vi "_Run Cycle Param.vi"(1 "Init (F)":bool) -> (0 "Finish Run?":bool)   [LabVIEW 2012]
uses:
  <vilib>/rvi/DataTransferAndStorage/Container/Common/niFpgaContainerGetUniqueNameForEmu.vi
  <vilib>/rvi/Memory/Memory_Emulation/niFpgaMemoryEmulationCacheClearOnFirstRun.vi
  <vilib>/rvi/Memory/Memory_Emulation/nirvimemoryEmulationManagerCache_MakeExclusive.vi
  <vilib>/rvi/Memory/Memory_Emulation/niFpgaMemoryEmulationValidateCache.vi
  <vilib>/rvi/Memory/Memory_Emulation/nirvimemoryEmulationManagerCache_ReleaseExclusive.vi
  <vilib>/rvi/Memory/Memory_Emulation/nirvimemoryEmulationManagerCache_InsertValue.vi
  <vilib>/Utility/error.llb/Clear Errors.vi
  <vilib>/rvi/Memory/Memory_Emulation/nirvimemoryEmulationManagerCache_GetValue.vi
  <vilib>/rvi/Emulation/niFpgaSctlEmulationGetInTimedLoop.vi
  <vilib>/rvi/Memory/Memory_Emulation/nirvimemoryEmulationManagerCache_SetValue.vi
  <vilib>/rvi/Emulation/niFpgaSctlEmulationResourceMgr.vi
  Instance           9 18Saved   _Run Cycle .vi
  <vilib>/rvi/DataTransferAndStorage/Container/XNode/niFpgaContainer.xnode
  <vilib>/rvi/Memory/Memory_Emulation/nirvimemoryEmulation.vi
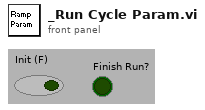
[diagram p1: front panel]
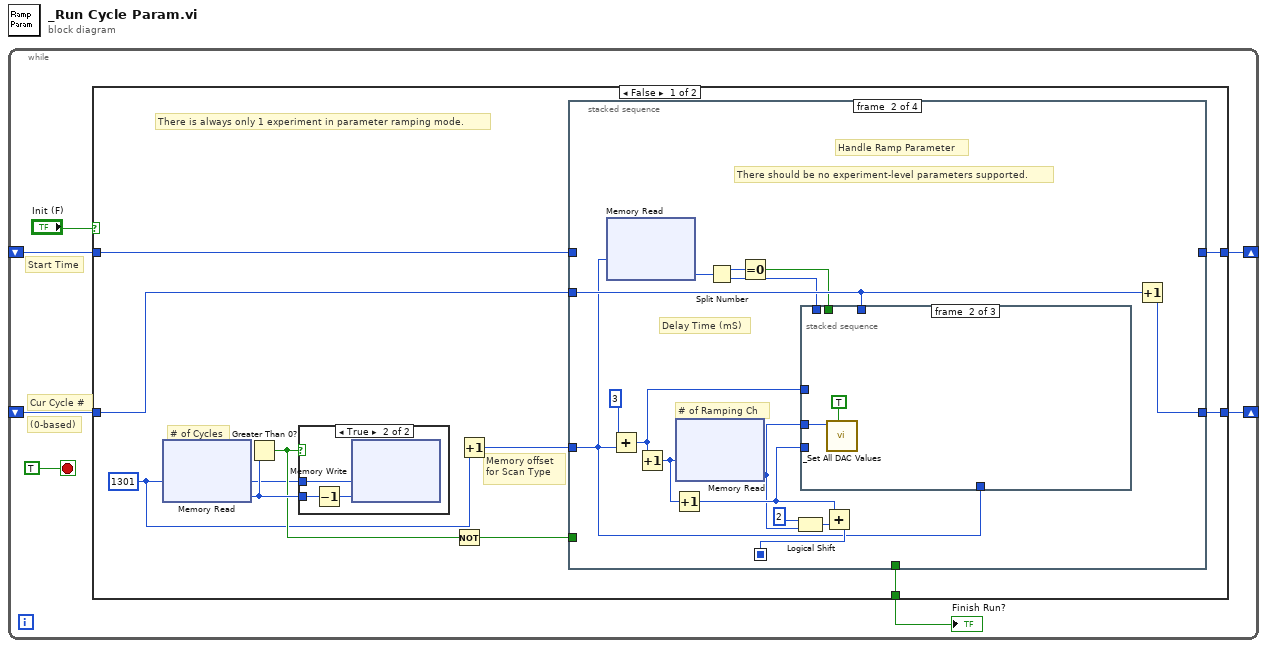
[diagram p0: block diagram]
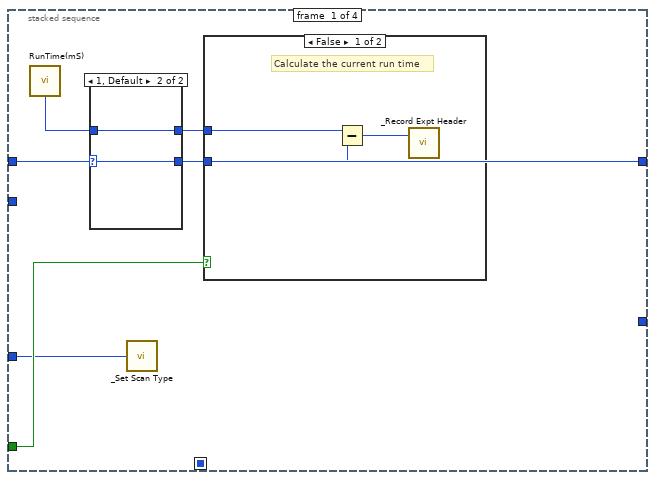
[diagram p3: hidden frame]
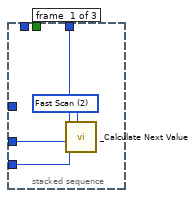
[diagram p6: hidden frame]
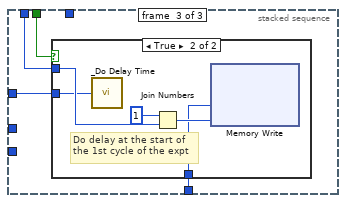
[diagram p7: hidden frame]
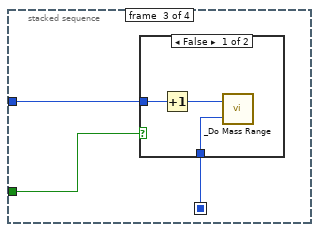
[diagram p9: hidden frame]
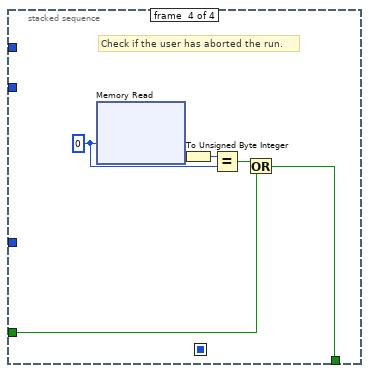
[diagram p11: hidden frame]
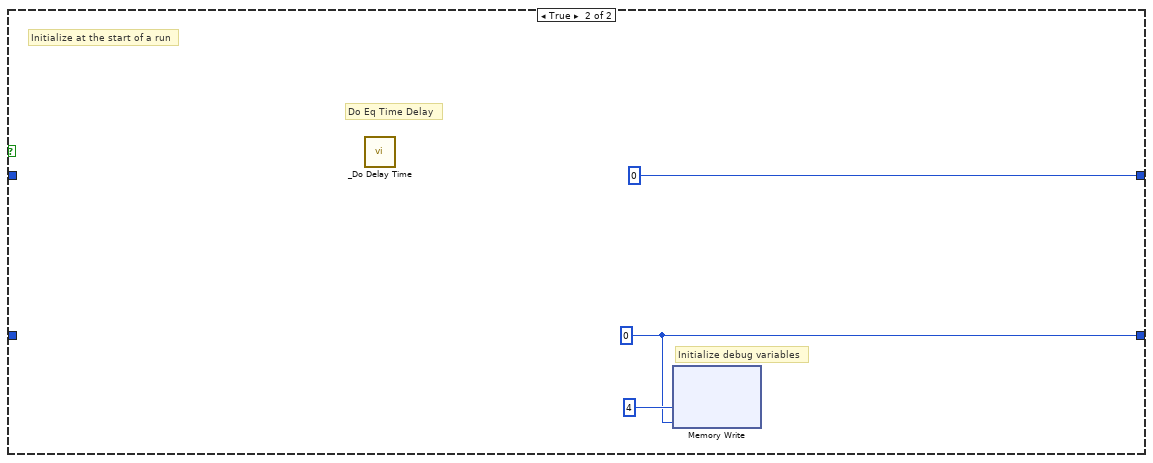
[diagram p12: hidden frame]
diagram:
  n1 = while {
    shift-right: [w6] -> _
    shift-left: _ -> [w5]
    shift-right: [w3] -> _
    shift-left: _ -> [w2]
    stop <- TRUE stop-if-true
    # "Cur Cycle #"
    # "(0-based)"
    # "Start Time"
    n2 = case shown="False" "Init (F)" {
      tunnel: [w8 u32 0 ("Tick Count(mSec)")] -> w6
      tunnel: w5 -> [w9 _]
      tunnel: [w15 w76] -> w3
      tunnel: w2 -> [w16 _]
      tunnel: [w10 _] -> w1
      frame False {
        w12 = u16 1301 ("Address")
        # "There is always only 1 experiment in parameter ramping mode."
        # "Memory offset\nfor Scan Type"
        # "# of Cycles"
        n3 = xnode ("Memory Read")("Address"=w12) -> ("Data"=w14:u32)  [unwired: 1 in, 1 out]
        n4 = Greater Than 0?(x=w14) -> (x > 0?=w13:bool)
        n5 = case shown="True" w13 {
          tunnel: w14 -> [_ w19]
          tunnel: w12 -> [_ w20]
          frame False {
          }
          frame True {
            n6 = Decrement(x=w19) -> (x-1=w18:u32)
            n7 = xnode ("Memory Write")("Address"=w20, "Data"=w18) -> ()  [unwired: 1 in, 1 out]
          }
        }
        n8 = Not(x=w13) -> (.not. x?=w11:bool)
        n9 = Increment(x=w12) -> (x+1=w17:u16)
        n10 = stacked-sequence {
          seq-local: [_ w39 _ _] -> [_ _ w65 _]
          tunnel: w16 -> [_ w45 _ _]
          tunnel: w11 -> [w26 _ w64 w70]
          tunnel: w17 -> [w25 w34 w63 _]
          tunnel: [_ w47 _ _] -> w15
          tunnel: [_ _ _ w69] -> w10
          tunnel: w9 -> [w24 _ _ _]
          tunnel: [w21 _ _ _] -> w8
          frame #0 {
            n11 = call "RunTime(mS)"() -> ("Tick Count(mSec)"=w23:u32)
            n12 = case shown="1, Default" w24 {
              selector: w24 -> [_ w29]
              tunnel: w23 -> [w27 w28]
              tunnel: [w27 w29] -> w21
              tunnel: [w27 w28] -> w22
              frame 0 {
              }
              frame 1, Default {
              }
            }
            n13 = call "_Set Scan Type.vi"("ScanType Offset"=w25) -> ()
            n14 = case shown="False" w26 {
              tunnel: w21 -> [w32 _]
              tunnel: w22 -> [w30 _]
              frame False {
                # "Calculate the current run time"
                n15 = Subtract(x=w30, y=w32) -> (x-y=w31:u32)
                n16 = call "_Record Expt Header.vi"("Run Time (mS)"=w31) -> ()  [unwired: 1 in, 1 out]
              }
              frame True {
              }
            }
          }
          frame #1 {
            # "There should be no experiment-level parameters supported."
            # "# of Ramping Ch"
            # "Delay Time (mS)"
            # "Handle Ramp Parameter"
            n17 = xnode ("Memory Read")("Address"=w34) -> ("Data"=w38:u32)  [unwired: 1 in, 1 out]
            n18 = Add(x=u8 3, y=w34) -> (x+y=w33:u16)
            n19 = Increment(x=w33) -> (x+1=w44:u16)
            n20 = Increment(x=w44) -> (x+1=w42:u16)
            n21 = xnode ("Memory Read")("Address"=w44) -> ("Data"=w41:u32)  [unwired: 1 in, 1 out]
            n22 = Split Number(x=w38) -> (hi(x)=w37:u16, lo(x)=w35:u16)
            n23 = Equal To 0?(x=w37) -> (x = 0?=w36:bool)
            n24 = Logical Shift(y=u8 2, x=w41) -> (x << y=w43:u32)
            n25 = stacked-sequence {
              tunnel: w41 -> [w51 w53 _]
              tunnel: w42 -> [w50 _ _]
              tunnel: w45 -> [w49 _ _]
              tunnel: w33 -> [_ _ w57]
              tunnel: w36 -> [_ _ w56]
              tunnel: w35 -> [_ _ w55]
              tunnel: w34 -> [_ _ w54]
              frame #0 {
                w48 = u8 2 items=["Positive", "Negative", "Fast Scan"] ("Polarity")
                n26 = call "_Calculate Next Value.vi"("Iteration#"=w49, "# of Ramping Ch"=w51, "Parameter Offset"=w50, "Polarity"=w48) -> ()  [unwired: 1 in, 1 out]
              }
              frame #1 {
                n27 = call "_Set All DAC Values.vi"("Record Values (F)"=TRUE, "# of Active Channels"=w53) -> ()  [unwired: 7 in]
              }
              frame #2 {
                n28 = case shown="True" w56 {
                  tunnel: w57 -> [_ w58]
                  tunnel: w55 -> [_ w60]
                  tunnel: w54 -> [_ w59]
                  frame False {
                  }
                  frame True {
                    # "Do delay at the start of \nthe 1st cycle of the expt"
                    n29 = call "_Do Delay Time.vi"("DelayTime Address"=w58) -> ()
                    n30 = Join Numbers(hi=u16 1, lo=w60) -> ((hi.lo)=w61:u32)
                    n31 = xnode ("Memory Write")("Address"=w59, "Data"=w61) -> ()  [unwired: 1 in, 1 out]
                  }
                }
              }
            }
            n32 = Add(x=w42, y=w43) -> (x+y=w39:u32)
            n33 = Increment(x=w45) -> (x+1=w47:u16)
          }
          frame #2 {
            n34 = case shown="False" w64 {
              tunnel: w65 -> [w68 _]
              tunnel: w63 -> [w67 _]
              frame False {
                n35 = Increment(x=w67) -> (x+1=w66:u16)
                n36 = call "_Do Mass Range.vi"("# of MR Offset"=w68, "Pause Time Offset"=w66) -> ()  [unwired: 2 out]
              }
              frame True {
              }
            }
          }
          frame #3 {
            w72 = u8 0 ("Address")
            # "Check if the user has aborted the run."
            n37 = xnode ("Memory Read")("Address"=w72) -> ("Data"=w74:u32)  [unwired: 1 in, 1 out]
            n38 = To Unsigned Byte Integer(number=w74) -> (unsigned 8bit integer=w73:u8)
            n39 = Equal?(x=w73, y=w72) -> (x = y?=w71:bool)
            n40 = Or(x=w71, y=w70) -> (x .or. y?=w69:bool)
          }
        }
      }
      frame True {
        w76 = u16 0 ("Data")
        # "Do Eq Time Delay"
        # "Initialize debug variables"
        # "Initialize at the start of a run"
        n41 = call "_Do Delay Time.vi"() -> ()  [unwired: 1 in]
        n42 = xnode ("Memory Write")("Address"=u8 4, "Data"=w76) -> ()  [unwired: 1 in, 1 out]
      }
    }
    "Finish Run?" <- w1
  }
